vi "FX_Config Set CL Values.vi"(6 "Send Cmd Timout(ms)":u32, 7 "SlotIdx":i32, 8 "Error":errorcluster, 9 "CL":T1={"Gains"={"P"=0.0, "I"=0.0, "D"=0.0, "F"=0.0}, "Error Allowed"={"High"=0.0, "Low"=0.0}, "I Zone"={"High"=0.0, "Low"=-1000.0}, "Max Out"={"FWD"=1.0, "REV"=-1.0}, "Max I Accu"={"High"=10.0, "Low"=-10.0}, "CL Ramp Rate (S)"=0.0} {"Max I Accu"."Low" format="%#.8f"; "Max I Accu"."High" format="%#.8f"; "Gains"."F" format="%#.8f"; "Gains"."D" format="%#.8f"; "Gains"."I" format="%#.8f"; "Gains"."P" format="%#.8f"; "Error Allowed"."Low" format="%#.8f"; "Error Allowed"."High" format="%#.8f"; "I Zone"."Low" format="%#.8f"; "I Zone"."High" format="%#.8f"; "Max Out"."REV" format="%.2f"; "Max Out"."FWD" format="%.2f"}, 11 "PhoenixMotorControlDevRef":T5) -> (0 "Error Out":errorcluster, 1 "CL Out":T1={"Gains"={"P"=0.0, "I"=0.0, "D"=0.0, "F"=0.0}, "Error Allowed"={"High"=0.0, "Low"=0.0}, "I Zone"={"High"=0.0, "Low"=-1000.0}, "Max Out"={"FWD"=1.0, "REV"=-1.0}, "Max I Accu"={"High"=10.0, "Low"=-10.0}, "CL Ramp Rate (S)"=0.0} {"Max I Accu"."Low" format="%#.8f"; "Max I Accu"."High" format="%#.8f"; "Gains"."F" format="%#.8f"; "Gains"."D" format="%#.8f"; "Gains"."I" format="%#.8f"; "Gains"."P" format="%#.8f"; "Error Allowed"."Low" format="%#.8f"; "Error Allowed"."High" format="%#.8f"; "I Zone"."Low" format="%#.8f"; "I Zone"."High" format="%#.8f"; "Max Out"."REV" format="%.2f"; "Max Out"."FWD" format="%.2f"}, 3 "PhoenixMotorControlDevRef Out":T5)   [LabVIEW 2020]
uses:
  Shared Code/TypeDefs/Cluster_PID Config.ctl
  Shared Code/TypeDefs/Cluster_PID Gains.ctl
  Shared Code/TypeDefs/Cluster_High-Low.ctl
  Shared Code/TypeDefs/Cluster_FWD  REV Values.ctl
  <vilib>/Rock Robotics/WPI/MotorControl/WPI_MotorControlDeviceRef.ctl
  <vilib>/Rock Robotics/WPI/MotorControl/WPI_MotorControlType.ctl
  <vilib>/Rock Robotics/SystemInterfaces/DIO/FPGA_DIOPWMChannel.ctl
  <vilib>/Rock Robotics/WPI/PWM/WPI_PWMDeadband.ctl
  <vilib>/Rock Robotics/SystemInterfaces/DIO/FPGA_DIOChannel.ctl
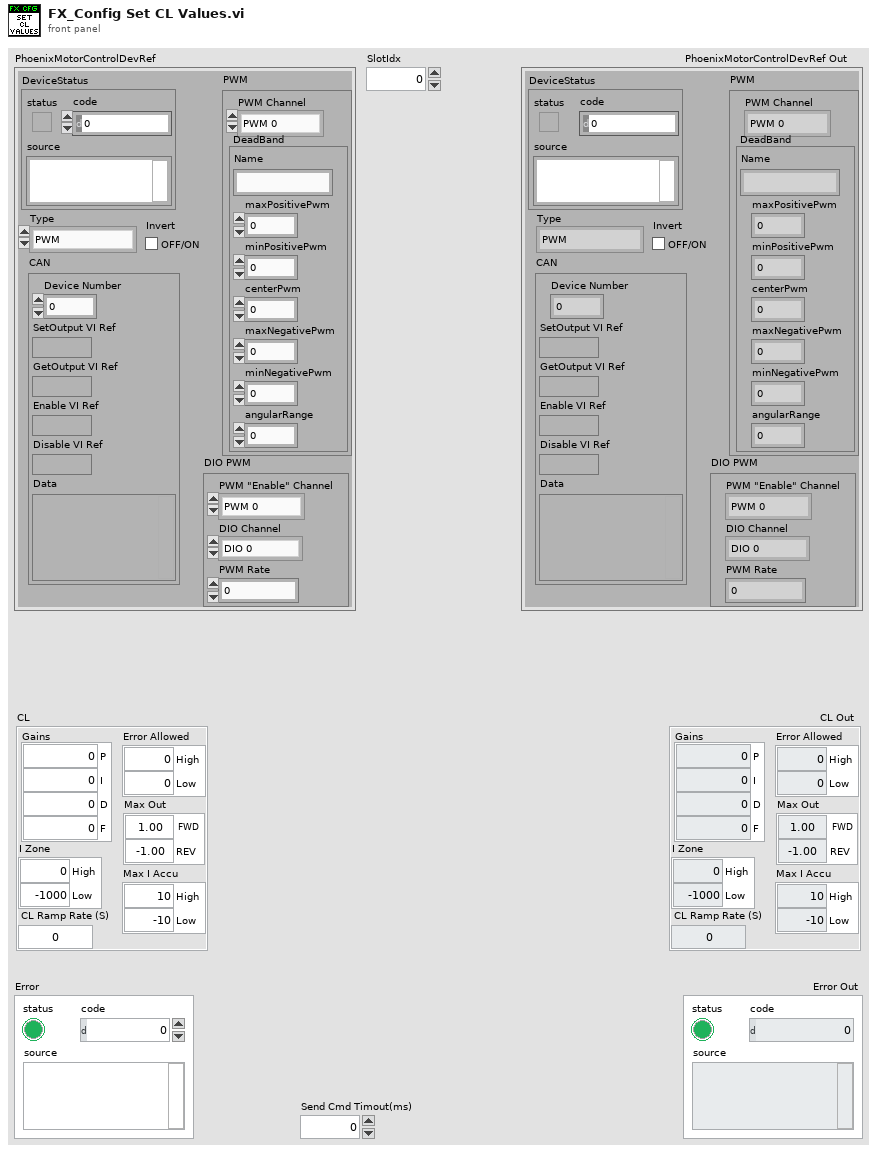
[diagram p1: front panel]
types:
  T1 = typedef "Cluster_PID Config.ctl" = cluster{"Gains":T2, "Error Allowed":T3, "I Zone":T3, "Max Out":T4, "Max I Accu":T3, "CL Ramp Rate (S)":dbl}
  T2 = typedef "Cluster_PID Gains.ctl" = cluster{"P":dbl, "I":dbl, "D":dbl, "F":dbl}
  T3 = typedef "Cluster_High-Low.ctl" = cluster{"High":dbl, "Low":dbl}
  T4 = typedef "Cluster_FWD  REV Values.ctl" = cluster{"FWD":dbl, "REV":dbl}
  T5 = typedef "WPI_MotorControlDeviceRef.ctl" = cluster{"DeviceStatus":errorcluster, "Type":T6, "PWM":cluster{"PWM Channel":T7, "DeadBand":T8}, "CAN":cluster{"Device Number":u8, "SetOutput VI Ref":variant, "GetOutput VI Ref":variant, "Enable VI Ref":variant, "Disable VI Ref":variant, "Data":variant}, "Invert":bool, "DIO PWM":cluster{"PWM \"Enable\" Channel":T7, "DIOChannel":T9, "PWM Rate":dbl}}
  T6 = typedef "WPI_MotorControlType.ctl" = enum16{"PWM", "CAN", "DIO PWM"}
  T7 = typedef "FPGA_DIOPWMChannel.ctl" = enum8{"PWM 0", "PWM 1", "PWM 2", "PWM 3", "PWM 4", "PWM 5", "PWM 6", "PWM 7", "PWM 8", "PWM 9", "PWM MXP 0", "PWM MXP 1", "PWM MXP 2", "PWM MXP 3", "PWM MXP 4", "PWM MXP 5", "PWM MXP 6", "PWM MXP 7", "PWM MXP 8", "PWM MXP 9", "Invalid"}
  T8 = typedef "WPI_PWMDeadband.ctl" = cluster{"Name":string, "maxPositivePwm":i32, "minPositivePwm":i32, "centerPwm":i32, "maxNegativePwm":i32, "minNegativePwm":i32, "angularRange":u16}
  T9 = typedef "FPGA_DIOChannel.ctl" = enum8{"DIO 0", "DIO 1", "DIO 2", "DIO 3", "DIO 4", "DIO 5", "DIO 6", "DIO 7", "DIO 8", "DIO 9", "DIO MXP 0", "DIO MXP 1", "DIO MXP 2", "DIO MXP 3", "DIO MXP 4", "DIO MXP 5", "DIO MXP 6", "DIO MXP 7", "DIO MXP 8", "DIO MXP 9", "DIO MXP 10", "DIO MXP 11", "DIO MXP 12", "DIO MXP 13", "DIO MXP 14", "DIO MXP 15", "SPI Port CS1", "SPI Port CS2", "SPI Port CS3", "SPI Port MISO", "SPI Port MOSI", "Invalid"}
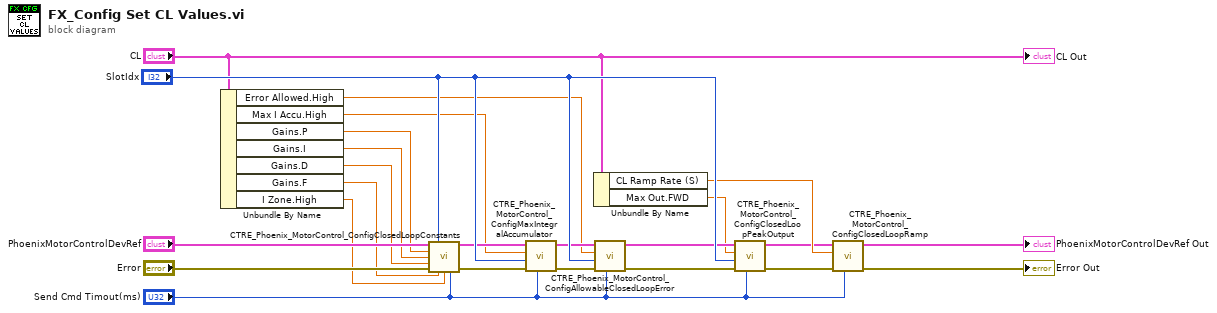
[diagram p0: block diagram]
diagram:
  n1 = Unbundle By Name("CL") -> ("Error Allowed.High"=w8:dbl, "Max I Accu.High"=w7:dbl, "Gains.P"=w13:dbl, "Gains.I"=w12:dbl, "Gains.D"=w11:dbl, "Gains.F"=w10:dbl, "I Zone.High"=w9:dbl)
  n2 = call <vilib>:"CTRE_Phoenix_MotorControl_ConfigClosedLoopConstants.vi"("PhoenixMotorControlDevRef"="PhoenixMotorControlDevRef", "slotIdx"="SlotIdx", "P"=w13, "I"=w12, "D"=w11, "error in (no error)"="Error", "F"=w10, "I Zone"=w9, "timeoutMs"="Send Cmd Timout(ms)") -> ("PhoenixMotorControlDevRef"=w14:T5, "error out"=w16:errorcluster)  [unwired: 5 in]
  n3 = call <vilib>:"CTRE_Phoenix_MotorControl_ConfigMaxIntegralAccumulator.vi"("timeoutMs"="Send Cmd Timout(ms)", "error in (no error)"=w16, "slotIdx"="SlotIdx", "Maximum Integral Accumulator Value"=w7, "PhoenixMotorControlDevRef"=w14) -> ("error out"=w17:errorcluster, "PhoenixMotorControlDevRef"=w15:T5)  [unwired: 5 in]
  n4 = Unbundle By Name("CL") -> ("CL Ramp Rate (S)"=w3:dbl, "Max Out.FWD"=w4:dbl)
  n5 = call <vilib>:"CTRE_Phoenix_MotorControl_ConfigAllowableClosedLoopError.vi"("timeoutMs"="Send Cmd Timout(ms)", "error in (no error)"=w17, "slotIdx"="SlotIdx", "allowableClosedLoopError"=w8, "PhoenixMotorControlDevRef"=w15) -> ("error out"=w5:errorcluster, "PhoenixMotorControlDevRef"=w6:T5)  [unwired: 5 in]
  n6 = call <vilib>:"CTRE_Phoenix_MotorControl_ConfigClosedLoopPeakOutput.vi"("timoutMs"="Send Cmd Timout(ms)", "error in (no error)"=w5, "slotIdx"="SlotIdx", "peakOutput"=w4, "PhoenixMotorControlDevRef"=w6) -> ("error out"=w1:errorcluster, "PhoenixMotorControlDevRef"=w2:T5)  [unwired: 5 in]
  n7 = call <vilib>:"CTRE_Phoenix_MotorControl_ConfigClosedLoopRamp.vi"("timeoutMs"="Send Cmd Timout(ms)", "error in (no error)"=w1, "secondsFromNeutralToFull"=w3, "PhoenixMotorControlDevRef"=w2) -> ("error out"=→"Error Out":errorcluster, "PhoenixMotorControlDevRef"=→"PhoenixMotorControlDevRef Out":T5)  [unwired: 6 in]
  "CL Out" <- "CL"
